vi "Test Get Output.vi"() -> ()   [LabVIEW 2016, in "Spectrum Recorder too.lvclass"]
uses:
  Spectrum Recorder too.lvclass
  Spectrum Recorder too.lvclass/Spectrum Recorder too.ctl
panel:
  out "size(s)":i32
  out "Output values out":dbl[](array[numeric])
  out "Waveform Graph":dbl[](graph)
  in  "Number of points":i32=100
  in  "User Configuration.Repeat (-1: forever)":i32=1
  in  "Output counter":i32
  in  "Records counter":i32
  in  "Output values in":dbl[](array[numeric])=[1.0, 2.0, 3.0, 4.0, 5.0, 6.0, 7.0, 8.0, 9.0, 10.0]
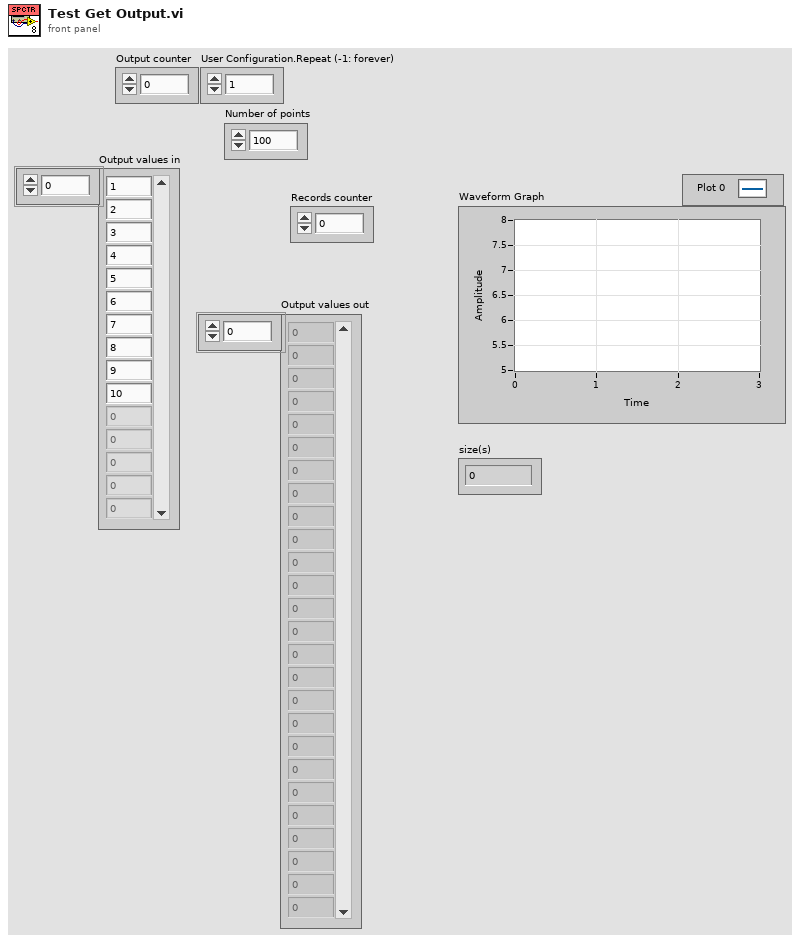
[diagram p1: front panel]
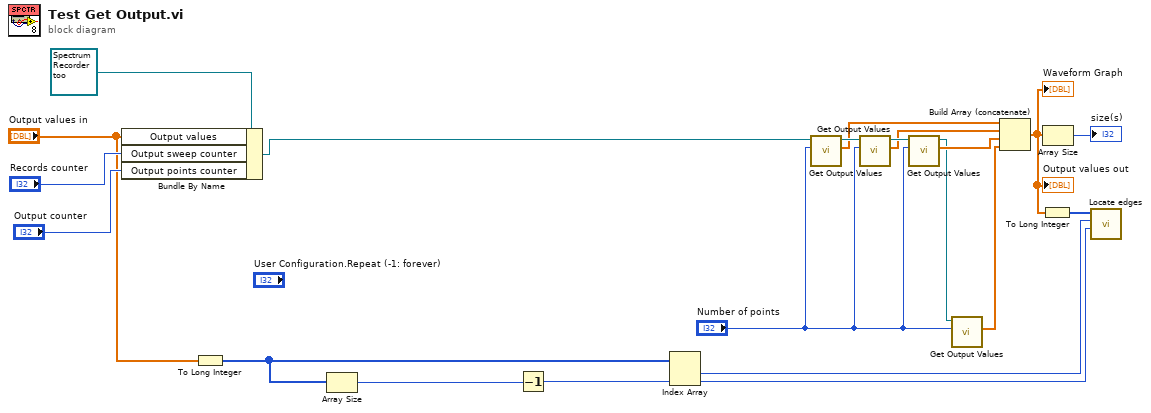
[diagram p0: block diagram]
diagram:
  n1 = Bundle By Name(cluster=refnum<class "Spectrum Recorder too.lvclass"> refnum ("Spectrum Recorder.lvclass"), "Output values"="Output values in", "Output sweep counter"="Records counter", "Output points counter"="Output counter") -> (w1:refnum<class "Spectrum Recorder too.lvclass">)
  n2 = To Long Integer(number="Output values in") -> (32bit integer=w3:i32[])
  n3 = Array Size(array=w3) -> (size(s)=w8:i32)
  n4 = Decrement(x=w8) -> (x-1=w7:i32)
  n5 = Index Array(array=w3, index #2=w7) -> (element #1=w6:i32, element #2=w5:i32)  [unwired: 1 in]
  n6 = call-dynamic "Get Output Values.vi"("Number of points"="Number of points", "Spectrum Recorder in"=w1) -> ("Output values"=w15:dbl[], "Spectrum Recorder out"=w17:refnum<class "Spectrum Recorder too.lvclass">)  [unwired: 7 in, 1 out]
  n7 = call-dynamic "Get Output Values.vi"("Number of points"="Number of points", "Spectrum Recorder in"=w17) -> ("Output values"=w14:dbl[], "Spectrum Recorder out"=w16:refnum<class "Spectrum Recorder too.lvclass">)  [unwired: 7 in, 1 out]
  n8 = call-dynamic "Get Output Values.vi"("Number of points"="Number of points", "Spectrum Recorder in"=w16) -> ("Output values"=w13:dbl[], "Spectrum Recorder out"=w12:refnum<class "Spectrum Recorder too.lvclass">)  [unwired: 7 in, 1 out]
  n9 = call-dynamic "Get Output Values.vi"("Number of points"="Number of points", "Spectrum Recorder in"=w12) -> ("Output values"=w10:dbl[])  [unwired: 7 in, 2 out]
  n10 = Build Array (concatenate)(w15, w14, w13, w10) -> (w9:dbl[])
  "Waveform Graph" <- w9
  "Output values out" <- w9
  n11 = To Long Integer(number=w9) -> (32bit integer=w2:i32[])
  n12 = Array Size(array=w9) -> (size(s)=→"size(s)":i32)
  n13 = call "Locate edges.vi"("Last value"=w5, "First value"=w6, "Values"=w2) -> ()  [unwired: 7 in, 2 out]
